vi "rcm_transform.vi"(10 "Tip and RCM":sgl[][](array[numeric]) format="%#_4p") -> (0 "Length":sgl, 2 "RCM transform":T1 format="%#_3f")   [LabVIEW 2013]
uses:
  <vilib>/Analysis/Matrix/Datatypes/RealMatrix.ctl
  norm_vec_single.vi
  <vilib>/Analysis/Matrix/Numeric/Conversions/Array To Matrix - RA.vi
  <vilib>/Analysis/Matrix/NI_Matrix.lvlib
panel:
  out "Theta XYZ":dbl[](array[numeric])
  # "Return transform generated from the Tip and RCM, taking the RCM as the origin.  When given the tool offsets, this computes the transform from RCM coordinates to output coordinates.  The two points only specify 5DOF, so the extra rotational DOF is used to force the rotation about z to zero."
  # "Distance from RCM to tip."
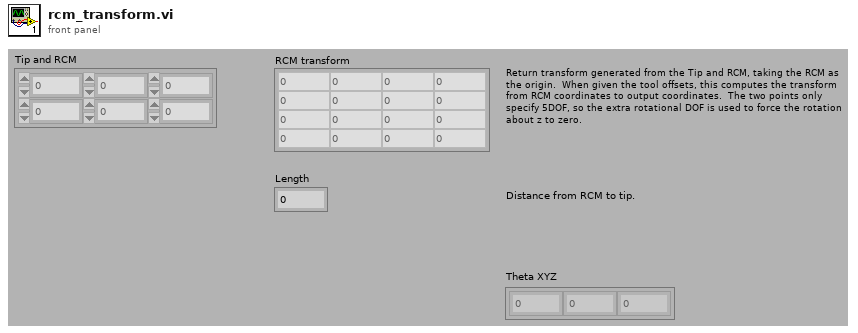
[diagram p1: front panel]
types:
  T1 = typedef "NI_Matrix.lvlib/RealMatrix.ctl" = dbl[][]
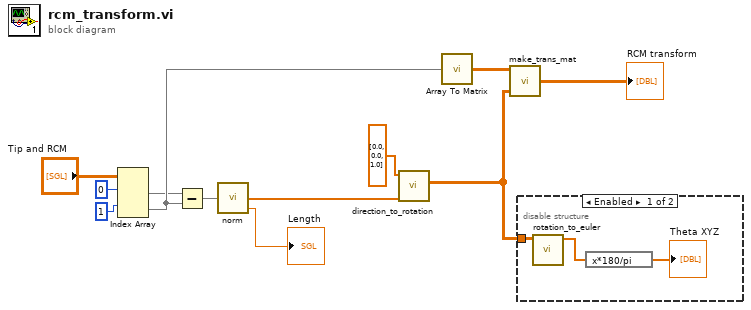
[diagram p0: block diagram]
diagram:
  n1 = Index Array(array="Tip and RCM", index (row) #1=0 ("index (row)"), index (row) #2=1 ("index (row)")) -> (element #1=w4:sgl[], element #2=w5:sgl[])  [unwired: 2 in]
  n2 = Subtract(x=w4, y=w5) -> (x-y=w10:sgl[])
  n3 = call-poly "norm.vi"("vector"=w10) -> ("magnitude"=→"Length":sgl, "normalized vector"=w3:sgl[])  [unwired: 3 in]
  n4 = call "direction_to_rotation.vi"("To"=w3, "From"=dbl[] [0.0, 0.0, 1.0]) -> ("Rotation"=w1:T1)  [unwired: 9 in]
  n5 = call-poly <vilib>:"Array To Matrix.vi"("Real 1D Array"=w5) -> ("Real Matrix (Column Vector)"=w9:T1)
  n6 = call "make_trans_mat.vi"("Rotation"=w1, "Translation"=w9) -> ("Transform"=→"RCM transform":T1)  [unwired: 3 in]
  n7 = disable-structure shown="Enabled" {
    disable-tunnel: w1 -> [w13 _]
    frame Enabled {
      n8 = call "rotation_to_euler.vi"("Rotation"=w13) -> ("Theta XYZ"=w15:dbl[])  [unwired: 10 in]
      n9 = expression code="x*180/pi"(w15) -> (→"Theta XYZ":dbl[])
    }
    frame Disabled {
    }
  }
